vi "ConvertTracepointsForServer.vi"(8 "error in (no error)":errorcluster, 10 "tracepoints":T4[](array[typedef]), 11 "config":T5) -> (0 "error out":errorcluster, 3 "message":T1)   [LabVIEW 2017, in "TracePointSynchronizer.lvlib"]
uses:
  <vilib>/addons/InsightCM/Devices/Shared/Common/TracePointSynchronizer/TracePointSynchronizer.lvlib
  <vilib>/addons/InsightCM/Devices/Shared/Common/TracePointSynchronizer/controls/config.ctl
  <vilib>/addons/InsightCM/Devices/Shared/Common/ServerComm/controls/ConnectionStatus.ctl
  <vilib>/addons/InsightCM/MessageBus/Base/controls/Message.ctl
  <vilib>/addons/InsightCM/MessageBus/Base/controls/MessageHeader.ctl
  <vilib>/addons/InsightCM/MessageBus/Base/controls/KeyValuePair.ctl
  <vilib>/addons/TraceLogger/controls/LogTracepoint.ctl
  <vilib>/addons/InsightCM/MessageBus/MessageLibrary/TraceLogger/controls/TraceLoggerStoreEntriesRoutedMessageBody.ctl
  <vilib>/addons/InsightCM/MessageBus/Base/controls/LogEntry.ctl
  <vilib>/addons/InsightCM/Devices/Shared/Common/ServerComm/ServerComm.lvlib
  <vilib>/addons/TraceLogger/TraceLogger.lvlib
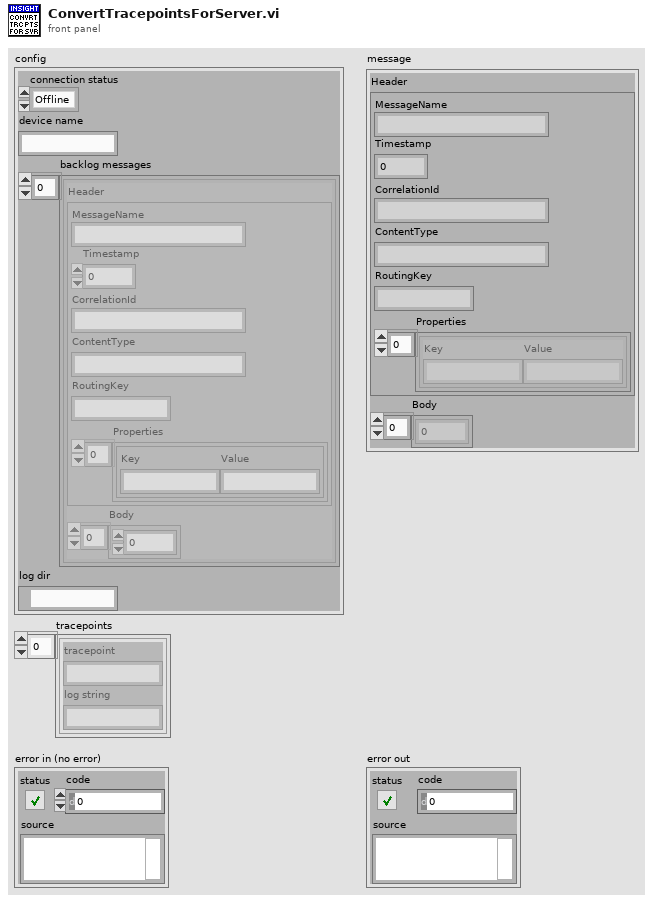
[diagram p1: front panel]
types:
  T1 = typedef "Message.ctl" = cluster{"Header":T2, "Body":u8[]}
  T2 = typedef "MessageHeader.ctl" = cluster{"MessageName":string, "Timestamp":i64, "CorrelationId":string, "ContentType":string, "RoutingKey":string, "Properties":T3[]}
  T3 = typedef "KeyValuePair.ctl" = cluster{"Key":string, "Value":string}
  T4 = typedef "TraceLogger.lvlib/LogTracepoint.ctl" = cluster{"tracepoint":string, "log string":string}
  T5 = typedef "TracePointSynchronizer.lvlib/config.ctl" = cluster{"connection status":T6, "device name":string, "backlog messages":T1[], "log dir":path}
  T6 = typedef "ServerComm.lvlib/ConnectionStatus.ctl" = enum16{"Offline", "NotAuthorized", "Online"}
  T7 = typedef "TraceLoggerStoreEntriesRoutedMessageBody.ctl" = cluster{"Entries":T8[]}
  T8 = typedef "LogEntry.ctl" = cluster{"ModuleName":string, "UnixTimestamp":i64, "TracePointName":string, "Text":string, "LogType":string}
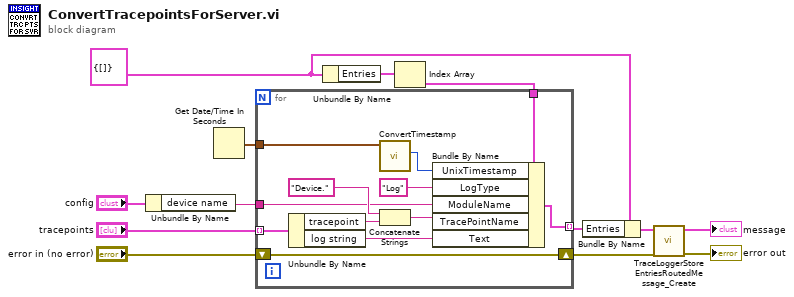
[diagram p0: block diagram]
diagram:
  w10 = T7 {"Entries"=[]} ("Body")
  n1 = Unbundle By Name("config") -> ("device name"=w13:string)
  n2 = Get Date/Time In Seconds() -> (seconds since 1Jan1904=w1:timestamp)
  n3 = Unbundle By Name(w10) -> ("Entries"=w8:T8[])
  n4 = Index Array(array=w8) -> (element=w9:T8)  [unwired: 1 in]
  n5 = for {
    tunnel: "tracepoints" -> [w25] mode=indexing
    shift-right: [w20] -> w4
    shift-left: "error in (no error)" -> [w20]
    tunnel: w9 -> [w22]
    tunnel: [w21] -> w11 mode=indexing
    tunnel: w13 -> [w17]
    tunnel: w1 -> [w14]
    n6 = Unbundle By Name(w25) -> ("tracepoint"=w23:string, "log string"=w19:string)
    n7 = call <vilib>:"ConvertTimestamp.vi"("Time Stamp"=w14) -> ("Timestamp out"=w15:i64)  [unwired: 10 in]
    n8 = Concatenate Strings("Device.", w23) -> (w18:string)
    n9 = Bundle By Name(cluster=w22, "UnixTimestamp"=w15, "LogType"="Log", "ModuleName"=w17, "TracePointName"=w18, "Text"=w19) -> (w21:T8)
  }
  n10 = Bundle By Name(cluster=w10, "Entries"=w11) -> (w5:T7)
  n11 = call <vilib>:"TraceLoggerStoreEntriesRoutedMessage_Create.vi"("error in (no error)"=w4, "TraceLoggerStoreEntriesRoutedMessage"=w5) -> ("error out"=→"error out":errorcluster, "Message"=→"message":T1)  [unwired: 8 in]
